vi "test_Set and Get 9423.vi"(8 "error in (no error)":errorcluster, 11 "TestCase in":refnum<class "Scan Engine Scripting API Custom Device Unit Tests.lvclass">) -> (0 "error out":errorcluster, 3 "TestCase out":refnum<class "Scan Engine Scripting API Custom Device Unit Tests.lvclass">)   [LabVIEW 2017, in "Scan Engine Scripting API Custom Device Unit Tests.lvclass"]
uses:
  Scan Engine Scripting API Custom Device Unit Tests.lvclass
  <vilib>/addons/_JKI Toolkits/VI Tester/TestCase.llb/TestCase.lvclass
  Scripting/Scan Engine Scripting.lvlib
  Type Defs/Main Settings.ctl
  Scan Engine Custom Device.lvlib
  Type Defs/Local Chassis Settings.ctl
  Scripting/Modules/NI 9423/NI 9423.lvclass
  C:/dev/github.com/debryant/niveristand-scan-engine-ethercat-custom-device/Custom Device Source/Scripting/Modules/Module/Module.lvclass
  C:/Program Files (x86)/National Instruments/LabVIEW 2017/vi.lib/addons/_JKI Toolkits/VI Tester/TestCase.llb/TestCase.lvclass
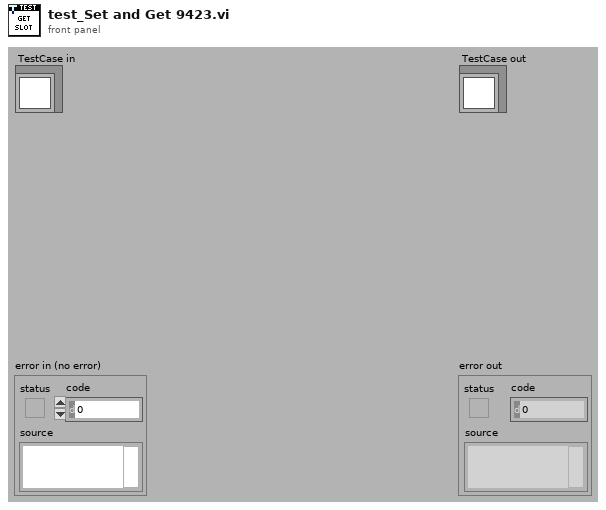
[diagram p1: front panel]
types:
  T1 = typedef "Scan Engine Custom Device.lvlib/Local Chassis Settings.ctl" = cluster{"name":string, "number of slots":i32}
  T2 = typedef "Scan Engine Custom Device.lvlib/Main Settings.ctl" = cluster{"sync to scan":bool, "scan engine decimation":u16, "delay after FPGA load (s)":u16}
  T3 = typedef "Custom Device API.lvlib/Custom Device Item Ref.ctl" = u64
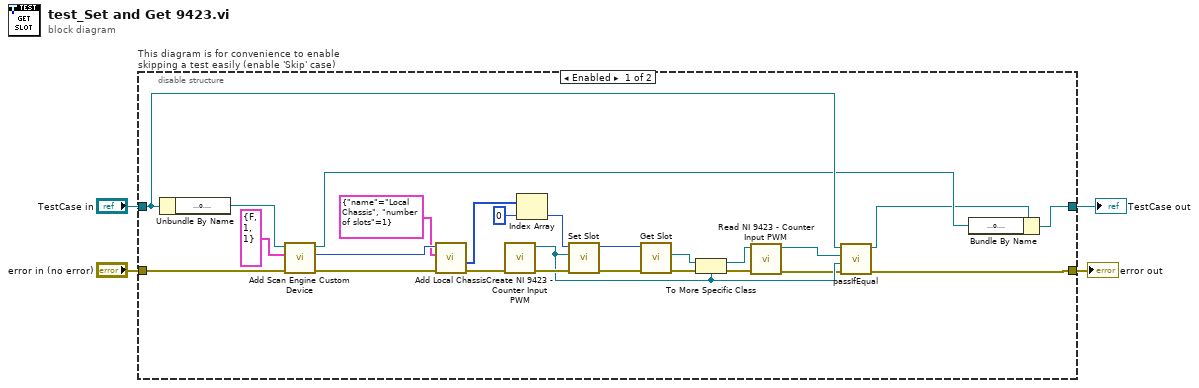
[diagram p0: block diagram]
diagram:
  n1 = disable-structure "This diagram is for convenience to enable skipping a test easily (enable 'Skip' case)" shown="Enabled" {
    disable-tunnel: "TestCase in" -> [w16 w33]
    disable-tunnel: [w20 w31] -> w1
    disable-tunnel: [w11 w32] -> w3
    disable-tunnel: "error in (no error)" -> [w28 w30]
    frame Enabled {
      n2 = Unbundle By Name(w16) -> ("target ref"=w27:refnum<k24>)
      n3 = call "Add Scan Engine Custom Device.vi"("error in"=w28, "settings"=T2 {"sync to scan"=FALSE, "scan engine decimation"=1, "delay after FPGA load (s)"=1}, "target in"=w27) -> ("error out"=w26:errorcluster, "scan engine custom device ref"=w25:T3, "target out"=w15:refnum<k24>)  [unwired: 6 in]
      n4 = call "Add Local Chassis.vi"("error in"=w26, "settings"=T1 {"name"="Local Chassis", "number of slots"=1}, "scan engine custom device ref in"=w25) -> ("error out"=w14:errorcluster, "slot refs"=w23:T3[])  [unwired: 4 in, 3 out]
      n5 = call "Create NI 9423 - Counter Input PWM.vi"("error in"=w14) -> ("error out"=w13:errorcluster, "module out"=w8:refnum<class "NI 9423.lvclass">)  [unwired: 9 in]
      n6 = Index Array(array=w23, index=0) -> (element=w22:T3)
      n7 = call "Set Slot.vi"("error in"=w13, "module"=w8, "slot ref in"=w22) -> ("error out"=w19:errorcluster, "slot ref out"=w5:T3)  [unwired: 7 in]
      n8 = call "Get Slot.vi"("error in"=w19, "slot ref in"=w5) -> ("error out"=w18:errorcluster, "module"=w17:refnum<class "Module.lvclass">)  [unwired: 6 in, 2 out]
      n9 = To More Specific Class(target class=w8, reference=w17, error in=w18) -> (specific class reference=w10:refnum<class "NI 9423.lvclass">, error out=w12:errorcluster)
      n10 = call "Read NI 9423 - Counter Input PWM.vi"("error in"=w12, "NI 9423 in"=w10) -> ("error out"=w7:errorcluster, "NI 9423 out"=w9:refnum<class "NI 9423.lvclass">)  [unwired: 7 in, 1 out]
      n11 = call-dynamic "passIfEqual.vi"("error in (no error)"=w7, "y"=w8, "x"=w9, "TestCase in"=w16) -> ("error out"=w11:errorcluster, "TestCase out"=w6:refnum<class "Scan Engine Scripting API Custom Device Unit Tests.lvclass">)  [unwired: 6 in]
      n12 = Bundle By Name(cluster=w6, "target ref"=w15) -> (w20:refnum<class "Scan Engine Scripting API Custom Device Unit Tests.lvclass">)
    }
    frame Disabled {
      # "skip test result while test is under development"
      n13 = call <vilib>:"skip.vi"("error in (no error)"=w30, "TestCase in"=w33) -> ("error out"=w32:errorcluster, "TestCase out"=w31:refnum<class "Scan Engine Scripting API Custom Device Unit Tests.lvclass">)  [unwired: 8 in]
    }
  }
  "error out" <- w3
  "TestCase out" <- w1
